vi "test.vi"(11 "Stimulator090724Scaffold in":refnum<class "Stimulator090724Scaffold.lvclass">) -> (3 "Stimulator090724Scaffold out":refnum<class "Stimulator090724Scaffold.lvclass">)   [LabVIEW 2010]
uses:
  main/labview_source/type_definitions/clusters/controls_refs.ctl
  GenericStimulator/GenericStimulator/trigger_enum.ctl
  GenericStimulator/GenericStimulator/GenericStimulator.lvclass
  common/clusters/plugin_specification.ctl
  Stimulator090724Scaffold.lvclass
  Clock/GenericClock/GenericClock/GenericClock.lvclass
panel:
  in  "pixel rate":dbl[unit]=80000.0
  in  "stop":bool
  in  "configuration name":string(combo)
  in  "create button":bool
  in  "stimulator component path":path
  in  "sweep button":bool
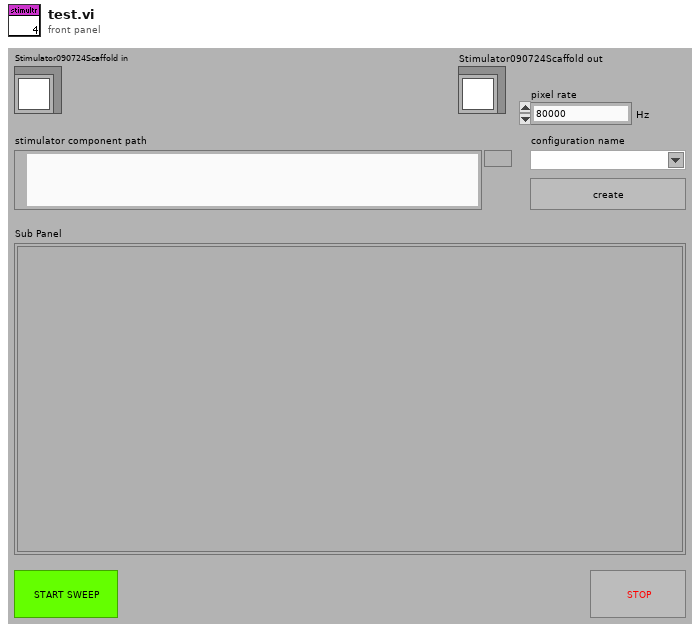
[diagram p1: front panel]
types:
  T1 = typedef "controls_refs.ctl" = cluster{"scan start button":refnum<vi>, "tabs":cluster{"main":refnum<vi>, "settings":refnum<vi>}, "subpanels":cluster{"imagingMode":refnum<vi>, "scanHead":refnum<vi>, "display":refnum<vi>, "experimentController":refnum<vi>, "instrument":refnum<vi>, "stage":refnum<vi>, "stimulator":refnum<vi>, "dataCollection":refnum<vi>, "analyser":refnum<vi>, "daq":refnum<vi>, "imageAssembler":refnum<vi>}, "drop-downs":cluster{"run mode":refnum<vi>, "imagingMode":refnum<vi>, "experimentalController":refnum<vi>, "objective":refnum<vi>}, "status lights":cluster{"experimentController":refnum<vi>, "imagingMode":refnum<vi>, "scanHead":refnum<vi>, "daq":refnum<vi>, "imageAssembler":refnum<vi>, "dataCollection":refnum<vi>, "display":refnum<vi>, "analyser":refnum<vi>, "stage":refnum<vi>, "stimulator":refnum<vi>, "instrument":refnum<vi>}, "message":refnum<vi>, "stimulator enabled?":refnum<vi>, "saving":cluster{"data folder path":refnum<vi>, "file base name":refnum<vi>, "notebook":refnum<vi>}, "progress bar":refnum<vi>, "update icon":refnum<vi>, "title":refnum<vi>, "main vi":refnum<vi>, "user":refnum<vi>, "exit_button":refnum<vi>, "CPU usage %":refnum<vi>}
  T2 = typedef "GenericStimulator.lvclass/trigger_enum.ctl" = enum16{"NULL", "initialise", "terminate", "start sweep", "stop sweep", "start continuous", "stop continuous"}
  T3 = typedef "plugin_specification.ctl" = cluster{"class path":string, "configuration":string, "label":string, "settings name":string}
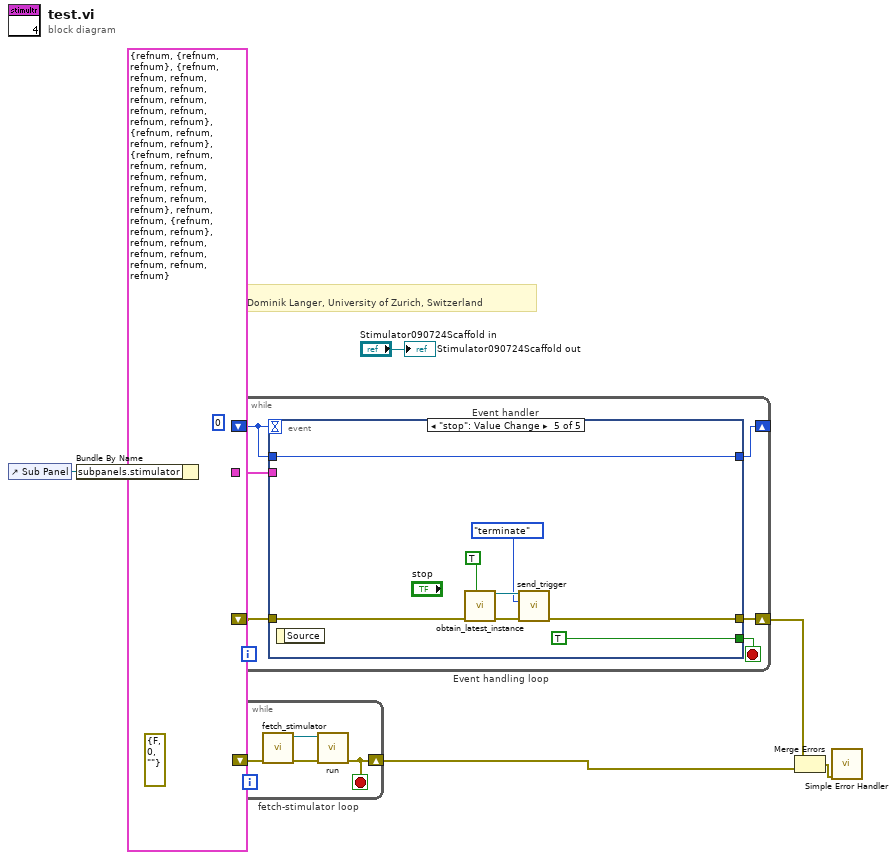
[diagram p0: block diagram]
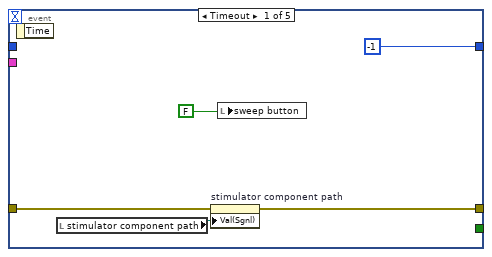
[diagram p2: hidden frame]
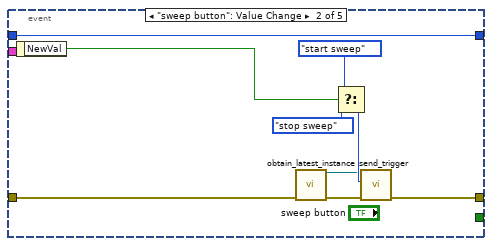
[diagram p3: hidden frame]
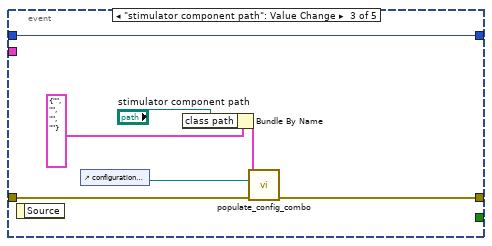
[diagram p4: hidden frame]
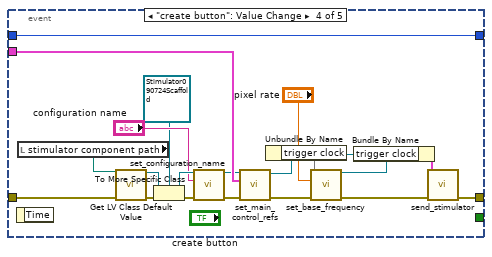
[diagram p5: hidden frame]
diagram:
  w8 = errorcluster {"status"=FALSE, "code"=0, "source"=""} ("error in (no error)")
  # "Authors: \n- created by: Dominik Langer, University of Zurich, Switzerland"
  n1 = control-ref of="Sub Panel"() -> (w2:refnum<vi>)
  n2 = Bundle By Name(cluster=T1 {"scan start button"=refnum, "tabs"={"main"=refnum, "settings"=refnum}, "subpanels"={"imagingMode"=refnum, "scanHead"=refnum, "display"=refnum, "experimentController"=refnum, "instrument"=refnum, "stage"=refnum, "stimulator"=refnum, "dataCollection"=refnum, "analyser"=refnum, "daq"=refnum, "imageAssembler"=refnum}, "drop-downs"={"run mode"=refnum, "imagingMode"=refnum, "experimentalController"=refnum, "objective"=refnum}, "status lights"={"experimentController"=refnum, "imagingMode"=refnum, "scanHead"=refnum, "daq"=refnum, "imageAssembler"=refnum, "dataCollection"=refnum, "display"=refnum, "analyser"=refnum, "stage"=refnum, "stimulator"=refnum, "instrument"=refnum}, "message"=refnum, "stimulator enabled?"=refnum, "saving"={"data folder path"=refnum, "file base name"=refnum, "notebook"=refnum}, "progress bar"=refnum, "update icon"=refnum, "title"=refnum, "main vi"=refnum, "user"=refnum, "exit_button"=refnum, "CPU usage %"=refnum} ("control references"), "subpanels.stimulator"=w2) -> (w1:T1)
  n3 = while "Event handling loop" {
    shift-right: [w12] -> w6
    shift-left: w8 -> [w15]
    shift-right: [w13] -> _
    shift-left: 0 -> [w14]
    tunnel: w1 -> [w10]
    stop <- w11 stop-if-true
    n4 = event "Event handler" shown="[4] \"stop\": Value Change" {
      selector: _ -> [_ _ _ _ _]
      dyn-events: _ -> [_ _ _ _ _]
      timeout: w14 -> [_ _ _ _ _]
      tunnel: w15 -> [w18 w24 w35 w54 w59]
      tunnel: w14 -> [_ w29 w36 w56 w64]
      tunnel: [-1 w29 w36 w56 w64] -> w13
      tunnel: [w17 w21 w33 w45 w58] -> w12
      tunnel: [_ _ _ _ TRUE] -> w11
      tunnel: w10 -> [_ _ _ w48 _]
      event Timeout {
        n5 = event-data() -> ()  [unwired: 2 out]
        n6 = local read "stimulator component path"() -> (w19:path)
        n7 = property on="stimulator component path" class="Path"(error in=w18, "Val(Sgnl)"=w19) -> (error out=w17:errorcluster)  [unwired: 1 in, 1 out]
        n8 = local write "sweep button"(FALSE) -> ()
      }
      event "sweep button": Value Change {
        n9 = event-data() -> ("NewVal"=w28:bool)  [unwired: 1 out]
        n10 = call "obtain_latest_instance.vi"("error in (no error)"=w24) -> ("error out"=w23:errorcluster, "GenericStimulator out"=w22:refnum<class "GenericStimulator.lvclass">)  [unwired: 1 in, 8 out]
        n11 = Select(t=trigger_enum."start sweep" ("trigger"), s=w28, f=trigger_enum."stop sweep") -> (s? t:f=w26:T2)
        n12 = call-dynamic "send_trigger.vi"("error in (no error)"=w23, "trigger"=w26, "GenericStimulator in"=w22) -> ("error out"=w21:errorcluster)  [unwired: 8 out]
      }
      event "stimulator component path": Value Change {
        n13 = event-data() -> ()  [unwired: 2 out]
        n14 = control-ref of="configuration name"() -> (w34:refnum<vi>)
        n15 = Bundle By Name(cluster=T3 {"class path"="", "configuration"="", "label"="", "settings name"=""} ("plug-in specification"), "class path"="stimulator component path") -> (w30:T3)
        n16 = call "populate_config_combo.vi"("error in (no error)"=w35, "combo-box reference"=w34, "plug-in specification"=w30) -> ("error out"=w33:errorcluster)  [unwired: 8 out]
      }
      event "create button": Value Change {
        n17 = event-data() -> ()  [unwired: 2 out]
        n18 = local read "stimulator component path"() -> (w55:path)
        n19 = call <vilib>:"Get LV Class Default Value.vi"("error in (no error)"=w54, "class path"=w55) -> ("error out"=w53:errorcluster, "object"=w51:refnum<class>)  [unwired: 8 out]
        n20 = To More Specific Class(target class=refnum<class "Stimulator090724Scaffold.lvclass"> refnum ("Stimulator090724Scaffold.lvclass"), reference=w51, error in=w53) -> (specific class reference=w50:refnum<class "Stimulator090724Scaffold.lvclass">, error out=w52:errorcluster)
        n21 = call-dynamic "set_configuration_name.vi"("error in (no error)"=w52, "configuration"="configuration name", "GenericPlugin.lvclass in"=w50) -> ("error out"=w47:errorcluster, "GenericPlugin.lvclass out"=w46:refnum<class "Stimulator090724Scaffold.lvclass">)  [unwired: 7 out]
        n22 = call-dynamic "set_main_control_refs.vi"("error in (no error)"=w47, "control references"=w48, "GenericPlugin.lvclass in"=w46) -> ("error out"=w41:errorcluster, "GenericPlugin.lvclass out"=w37:refnum<class "Stimulator090724Scaffold.lvclass">)  [unwired: 7 out]
        n23 = Unbundle By Name(w37) -> ("trigger clock"=w42)
        n24 = call-dynamic "set_base_frequency.vi"("error in (no error)"=w41, "base frequency"="pixel rate", "GenericClock.lvclass in"=w42) -> ("error out"=w40:errorcluster, "GenericClock.lvclass out"=w39:refnum<class "GenericClock.lvclass">)  [unwired: 7 out]
        n25 = Bundle By Name(cluster=w37, "trigger clock"=w39) -> (w38:cluster{})
        n26 = call-dynamic "send_stimulator.vi"("error in (no error)"=w40, "GenericStimulator in"=w38) -> ("error out"=w45:errorcluster)  [unwired: 9 out]
      }
      event "stop": Value Change {
        n27 = event-data() -> ()  [unwired: 2 out]
        n28 = call "obtain_latest_instance.vi"("quick, but maybe outdated?"=TRUE, "error in (no error)"=w59) -> ("error out"=w61:errorcluster, "GenericStimulator out"=w62:refnum<class "GenericStimulator.lvclass">)  [unwired: 8 out]
        n29 = call-dynamic "send_trigger.vi"("error in (no error)"=w61, "trigger"=trigger_enum."terminate", "GenericStimulator in"=w62) -> ("error out"=w58:errorcluster)  [unwired: 8 out]
      }
    }
  }
  n30 = while "fetch-stimulator loop" {
    shift-right: [w65] -> w5
    shift-left: w8 -> [w68]
    stop <- w65 stop-if-true
    n31 = call "fetch_stimulator.vi"("error in (no error)"=w68) -> ("error out"=w67:errorcluster, "GenericStimulator out"=w66:refnum<class "GenericStimulator.lvclass">)  [unwired: 9 out]
    n32 = call-dynamic "run.vi"("error in (no error)"=w67, "GenericStimulator in"=w66) -> ("error out"=w65:errorcluster)  [unwired: 9 out]
  }
  n33 = Merge Errors(w6, w5) -> (w7:errorcluster)
  n34 = call <vilib>:"Simple Error Handler.vi"("error in (no error)"=w7) -> ()  [unwired: 1 in, 8 out]
  "Stimulator090724Scaffold out" <- "Stimulator090724Scaffold in"
